vi "un 2.vi"() -> ()   [LabVIEW 2018]
panel:
  out "CARRY":bool
  out "SUM":bool
  in  "B":bool
  in  "A":bool
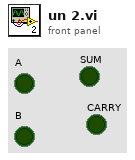
[diagram p1: front panel]
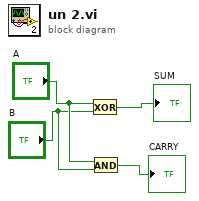
[diagram p0: block diagram]
diagram:
  n1 = Exclusive Or(1:"B", 2:"A") -> (0:→"SUM":bool)
  n2 = And(x="A", y="B") -> (x .and. y?=→"CARRY":bool)
